vi "Initialization.vi"(8 "error in (no error)":errorcluster, 9 "baud rate":u32=9600, 10 "VISA Resouce":string, 11 "Serial in":refnum<class "Serial.lvclass">) -> (0 "error out":errorcluster, 3 "Serial out":refnum<class "Serial.lvclass">)   [LabVIEW 2019, in "Serial.lvclass"]
uses:
  Serial.lvclass
  Serial.lvclass/Serial.ctl
  <vilib>/Instr/_visa.llb/VISA Configure Serial Port (Instr).vi
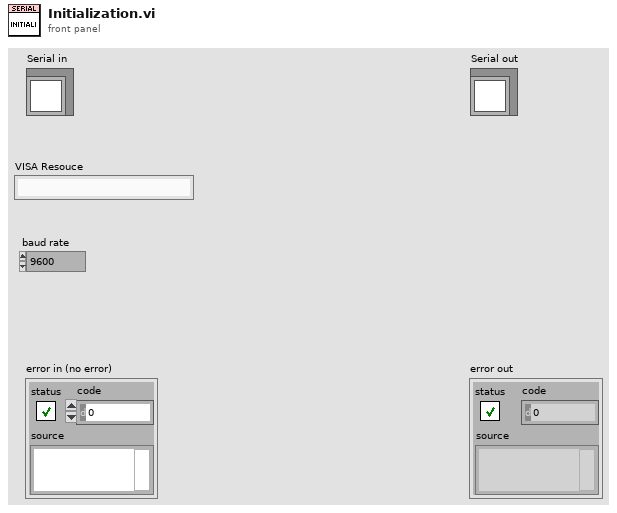
[diagram p1: front panel]
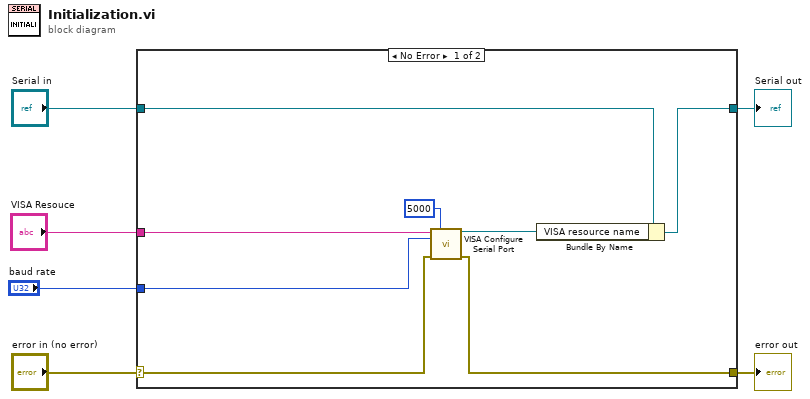
[diagram p0: block diagram]
diagram:
  n1 = case shown="No Error" "error in (no error)" {
    selector: "error in (no error)" -> [w13 w16]
    tunnel: [w12 w16] -> w5
    tunnel: [w10 w15] -> w3
    tunnel: "Serial in" -> [w11 w15]
    tunnel: "VISA Resouce" -> [w8 _]
    tunnel: "baud rate" -> [w7 _]
    frame No Error {
      n2 = call-poly "VISA Configure Serial Port"("VISA resource name"=w8, "timeout (10sec)"=u32 5000, "baud rate (9600)"=w7, "error in (no error)"=w13) -> ("VISA resource name out"=w9:refnum<visa-resource-name>, "error out"=w12:errorcluster)  [unwired: 6 in, 4 out]
      n3 = Bundle By Name(cluster=w11, "VISA resource name"=w9) -> (w10:refnum<class "Serial.lvclass">)
    }
    frame Error {
    }
  }
  "error out" <- w5
  "Serial out" <- w3
